vi "Convert to Legacy Error Cluster.vi"(11 "error in":errorcluster) -> (3 "error out":errorcluster)   [LabVIEW 2020, in "Multi Error Cluster.lvlib"]
doc: "Converts an error cluster from JSON encoded format to legacy format."
uses:
  <vilib>/MultiError/TokenizeJSON/Multi Error Cluster.lvlib
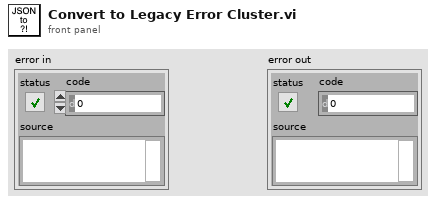
[diagram p1: front panel]
types:
  T1 = typedef "Multi Error Cluster.lvlib/JSON Token Values.ctl" = enum32{"array begin", "array end", "object begin", "object end", "value", "invalid", "name"}
  T2 = typedef "Multi Error Cluster.lvlib/JSON Token Descriptor.ctl" = cluster{"match string":string, "raw token type":T3, "byte offset ":i32}
  T3 = typedef "Multi Error Cluster.lvlib/JSON Raw Token Values.ctl" = enum32{"{", "}", "[", "]", ",", ":", "\"", "number", "string", "true", "false", "null", "invalid"}
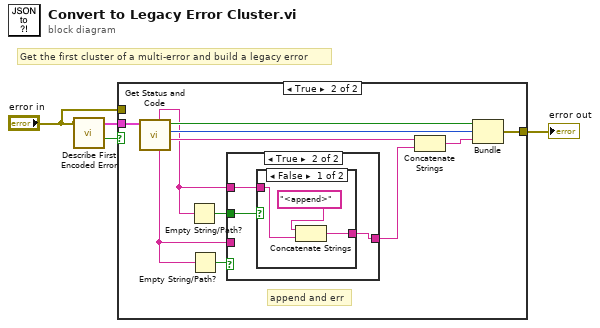
[diagram p0: block diagram]
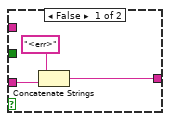
[diagram p3: hidden frame]
diagram:
  # "Get the first cluster of a multi-error and build a legacy error"
  n1 = call <vilib>:"Describe First Encoded Error.vi"("error in"="error in") -> ("encoded"=w2:bool, "tokens"=w3:cluster{"token type":T1, T2}[])  [unwired: 9 in]
  n2 = case shown="True" w2 {
    tunnel: w3 -> [_ w13]
    tunnel: [w5 w14] -> w4
    tunnel: "error in" -> [w5 _]
    frame False {
    }
    frame True {
      # "append and err"
      n3 = call <vilib>:"Get Status and Code.vi"("tokens"=w13) -> ("source"=w12:string, "code"=w15:i32, "status"=w16:bool, "substitute"=w9:string, "additional"=w7:string)  [unwired: 6 in]
      n4 = Empty String/Path?(string/path=w7) -> (empty?=w8:bool)
      n5 = Empty String/Path?(string/path=w9) -> (empty?=w10:bool)
      n6 = case shown="True" w10 {
        tunnel: w9 -> [w18 _]
        tunnel: [w17 w20] -> w6
        tunnel: w8 -> [_ w22]
        tunnel: w7 -> [_ w21]
        frame False {
          n7 = Concatenate Strings("<err>", w18) -> (w17:string)
        }
        frame True {
          n8 = case shown="False" w22 {
            tunnel: w21 -> [w24 _]
            tunnel: [w23 _] -> w20
            frame False {
              n9 = Concatenate Strings("<append>", w24) -> (w23:string)
            }
            frame True {
            }
          }
        }
      }
      n10 = Concatenate Strings(w12, w6) -> (w11:string)
      n11 = Bundle("status"=w16, "code"=w15, w11) -> (w14:cluster{"status":bool, "code":i32, string})  [unwired: 1 in]
    }
  }
  "error out" <- w4
